vi "Refill Syringe.vi"(8 "error in (no error)":errorcluster, 9 "auto_switch_valve":bool=TRUE, 10 "flow_rate_uL_s":dbl=200.0, 11 "Wait for pump":bool) -> (0 "error out":errorcluster)   [LabVIEW 2018, in "cetoni.lvlib" / "cetoni.lvclass"]
uses:
  cetoni.lvclass
  Resources/GLOBAL/GLOBAL Time-critical.vi
  <userlib>/QmixLib/QmixLib.lvlib
  Program Files/cetoni/QmixSDK/lib/labview/labbCAN_Pump_API/labbCAN_Pump_API.lvlib
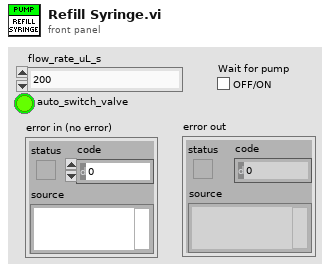
[diagram p1: front panel]
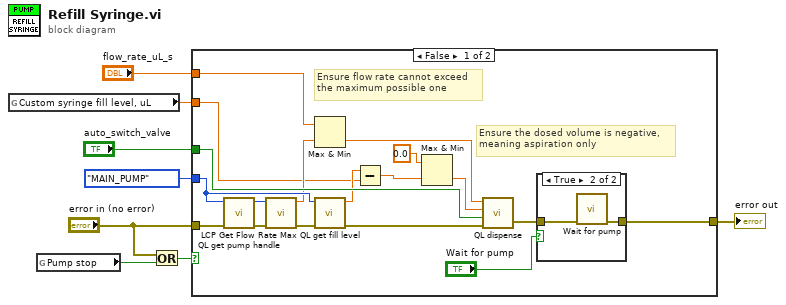
[diagram p0: block diagram]
diagram:
  n1 = global read "GLOBAL Time-critical.vi" "Custom syringe fill level, uL"() -> (w4:dbl)
  n2 = global read "GLOBAL Time-critical.vi" "Pump stop"() -> (w2:bool)
  n3 = Or(x="error in (no error)", y=w2) -> (x .or. y?=w1:bool)
  n4 = case shown="False" w1 {
    tunnel: [w10 w30] -> w8
    tunnel: enum16{"MAIN_PUMP"}."MAIN_PUMP" ("pump") -> [w22 _]
    tunnel: "auto_switch_valve" -> [w25 _]
    tunnel: "flow_rate_uL_s" -> [w20 _]
    tunnel: w4 -> [w18 _]
    tunnel: "error in (no error)" -> [w9 w30]
    frame False {
      # "Ensure the dosed volume is negative,\nmeaning aspiration only"
      # "Ensure flow rate cannot exceed\nthe maximum possible one"
      n5 = call <userlib>:"QL get pump handle.vi"("error in (no error)"=w9, "pump"=w22) -> ("error out"=w26:errorcluster, "pump handle"=w16:u64)  [unwired: 8 in]
      n6 = call "LCP Get Flow Rate Max.vi"("error in (no error)"=w26, "Pump Handle"=w16) -> ("error out"=w23:errorcluster, "Maximum Flow Rate"=w21:dbl)  [unwired: 8 in]
      n7 = Max & Min(x=w20, y=w21) -> (min(x,y)=w24:dbl)  [unwired: 1 out]
      n8 = call <userlib>:"QL get fill level.vi"("error in (no error)"=w23, "pump"=w22) -> ("error out"=w17:errorcluster, "Fill level, uL"=w19:dbl)  [unwired: 8 in]
      n9 = Subtract(x=w19, y=w18) -> (x-y=w13:dbl)
      n10 = Max & Min(x=0.0, y=w13) -> (min(x,y)=w14:dbl)  [unwired: 1 out]
      n11 = call <userlib>:"QL dispense.vi"("error in (no error)"=w17, "auto_switch_valve"=w25, "volume_uL"=w14, "flow_rate_uL_s"=w24) -> ("error out"=w11:errorcluster)  [unwired: 3 in]
      n12 = case shown="True" "Wait for pump" {
        tunnel: w11 -> [w27 w29]
        tunnel: [w27 w28] -> w10
        frame False {
        }
        frame True {
          n13 = call "Wait for pump.vi"("error in (no error)"=w29) -> ("error out"=w28:errorcluster)  [unwired: 10 in]
        }
      }
    }
    frame True {
    }
  }
  "error out" <- w8
